vi "TCP-IP Mgr.Core.vi"(9 "Q Message Templates":T3={"Status.Q.Msg"={"Cmd"="Task", "Sub"="TCP-IP Connect Event", "Data1"=variant, "Data2"=variant}, "Rcv.Q.Msg"={"Cmd"="Task", "Sub"="TCP-IP Rcv", "Data1"=variant, "Data2"=variant}}, 10 "Config":T5={"IP"="127.0.0.1", "Port"=8500, "Listener"=FALSE, "Enable"=FALSE}, 11 "Module Config":T1={"Name"="TCP-IP Mgr", "Parent Q"=refnum, "Is Child?"=FALSE, "Index"=0, "Dirs"={"Root"=path "", "Config"=path "", "Logs"=path "", "Reports"=path "", "App Data"=path ""}, "Simulate"=FALSE, "SimCtrl"=refnum}) -> ()   [LabVIEW 2024, in "EQMF.lvlib" / "TCP-IP.lvlib"]
uses:
  TCP-IP.lvlib
  Module/Module Config.ctl
  Queues/Q.Element.ctl
  Module/Module.Working Dirs.ctl
  TCP-IP Mgr.Cluster - Q Message Templates.ctl
  TCP-IP Mgr.Config.ctl
  Module/Window/Window.Task, Action.ctl
  Strings/TextBoxLogCtrlMgr/TextBoxLogCtrlMgr.lvclass
  <vilib>/Utility/error.llb/Trim Whitespace One-Sided.vi
  Queues/Queue Utils.lvlib
  Module/Module Utils.lvlib
  Controls/Controls.lvlib
  Event Log/Event Log.lvlib
  Status/Status Utils.lvlib
panel:
  in  "Main Tab":enum32{"Operate", "Maint"}(tab)
  out "IP":string
  out "Status":string
  in  "Auto Scroll":bool
  out "Log":string
  in  "Clear":bool
  in  "Maint":bool
  out "Port":u16=8500
  in  "Show Block Diagram":bool
  in  "Leave Maint":bool
  in  "Exit":bool
  in  "Cnct Timeout":i32=1000
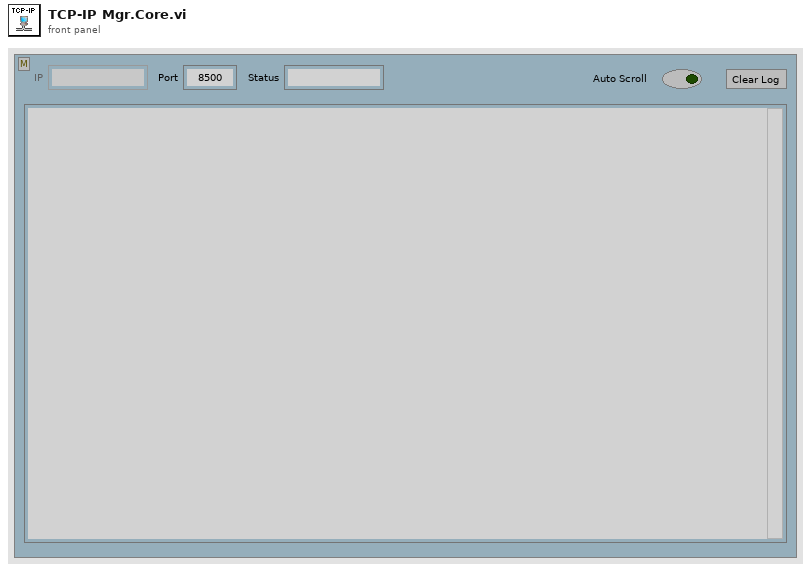
[diagram p1: front panel]
types:
  T1 = typedef "EQMF.lvlib/Module Utils.lvlib/Module Config.ctl" = cluster{"Name":string, "Parent Q":refnum<queue>, "Is Child?":bool, "Index":i32, "Dirs":T2, "Simulate":bool, "SimCtrl":refnum<vi>}
  T2 = typedef "EQMF.lvlib/Module Utils.lvlib/Module.Working Dirs.ctl" = cluster{"Root":path, "Config":path, "Logs":path, "Reports":path, "App Data":path}
  T3 = typedef "EQMF.lvlib/TCP-IP.lvlib/TCP-IP Mgr.Cluster - Q Message Templates.ctl" = cluster{"Status.Q.Msg":T4, "Rcv.Q.Msg":T4}
  T4 = typedef "EQMF.lvlib/Queue Utils.lvlib/Q.Element.ctl" = cluster{"Cmd":string, "Sub":string, "Data1":variant, "Data2":variant}
  T5 = typedef "EQMF.lvlib/TCP-IP.lvlib/TCP-IP Mgr.Config.ctl" = cluster{"IP":string, "Port":u16, "Listener":bool, "Enable":bool}
  T6 = typedef "EQMF.lvlib/Module Utils.lvlib/Module Sys Info.ctl" = cluster{"Main Q":refnum<queue>, "Exe":bool, "SW Rev":T7, "Self Ref":refnum<vi>, "Main Tab":refnum<vi>, "Pane":refnum<vi>, "Stop":cluster{"Ref":refnum<event-registration>, "Event":refnum<user-event>}, "Cfg":T1, "Services":cluster{"Name":string, "vi ref":refnum<vi>}[], "Menu Ref":refnum<k9>, "CtrlStates":refnum<class "Class.SaveCtrls.lvclass">, "Docs":cluster{"Tags":string[], "Paths":path[]}, "Log":refnum<class "Event Notification.lvclass">, "Test Controls":refnum<vi>[], "Child Modules":cluster{"Name":string, "vi ref":refnum<vi>}[], "SW Items":string[][], "AppData":refnum<class "Class.AppData.lvclass">, "Subscriptions":refnum<class "Subscription.lvclass">, "Module Config Ref":refnum<vi>}
  T7 = typedef "EQMF.lvlib/Module Utils.lvlib/Module.SW Version Info.ctl" = cluster{"AppName":string, "Company":string, "Version":string, "Description":string, "PN":string}
  T8 = typedef "EQMF.lvlib/Module Utils.lvlib/Window.Task, Action.ctl" = enum16{"Resize()", "Show Panel(Bool)", "Show Scroll Bars(Bool)", "Dock to SubPanel(SubPanel Ref)", "Undock from SubPanel()", "Return to SubPanel()", "Go To Maint Tab()", "Show Maint Tab(Bool)", "Open Block Diagram()"}
  T9 = enum16{"Top Left", "Top Right", "Bottom Left", "Bottom Right"}
  T10 = cluster{"Log":string, "Status.Q.Msg":T4, "LogMgr":refnum<class "TextBoxLogCtrlMgr.lvclass">}
  T11 = typedef "EQMF.lvlib/Status Utils.lvlib/Status.ErrorAction - Exit, Reset, Ignore.ctl" = enum16{"Exit", "Reset", "Ignore"}
  T12 = enum8{"Enabled", "Disabled", "Disabled and Grayed Out"}
  T13 = cluster{"Connected":bool, "TCPIP ID":refnum<k5>, "Config":T5, "QMsgs":T3}
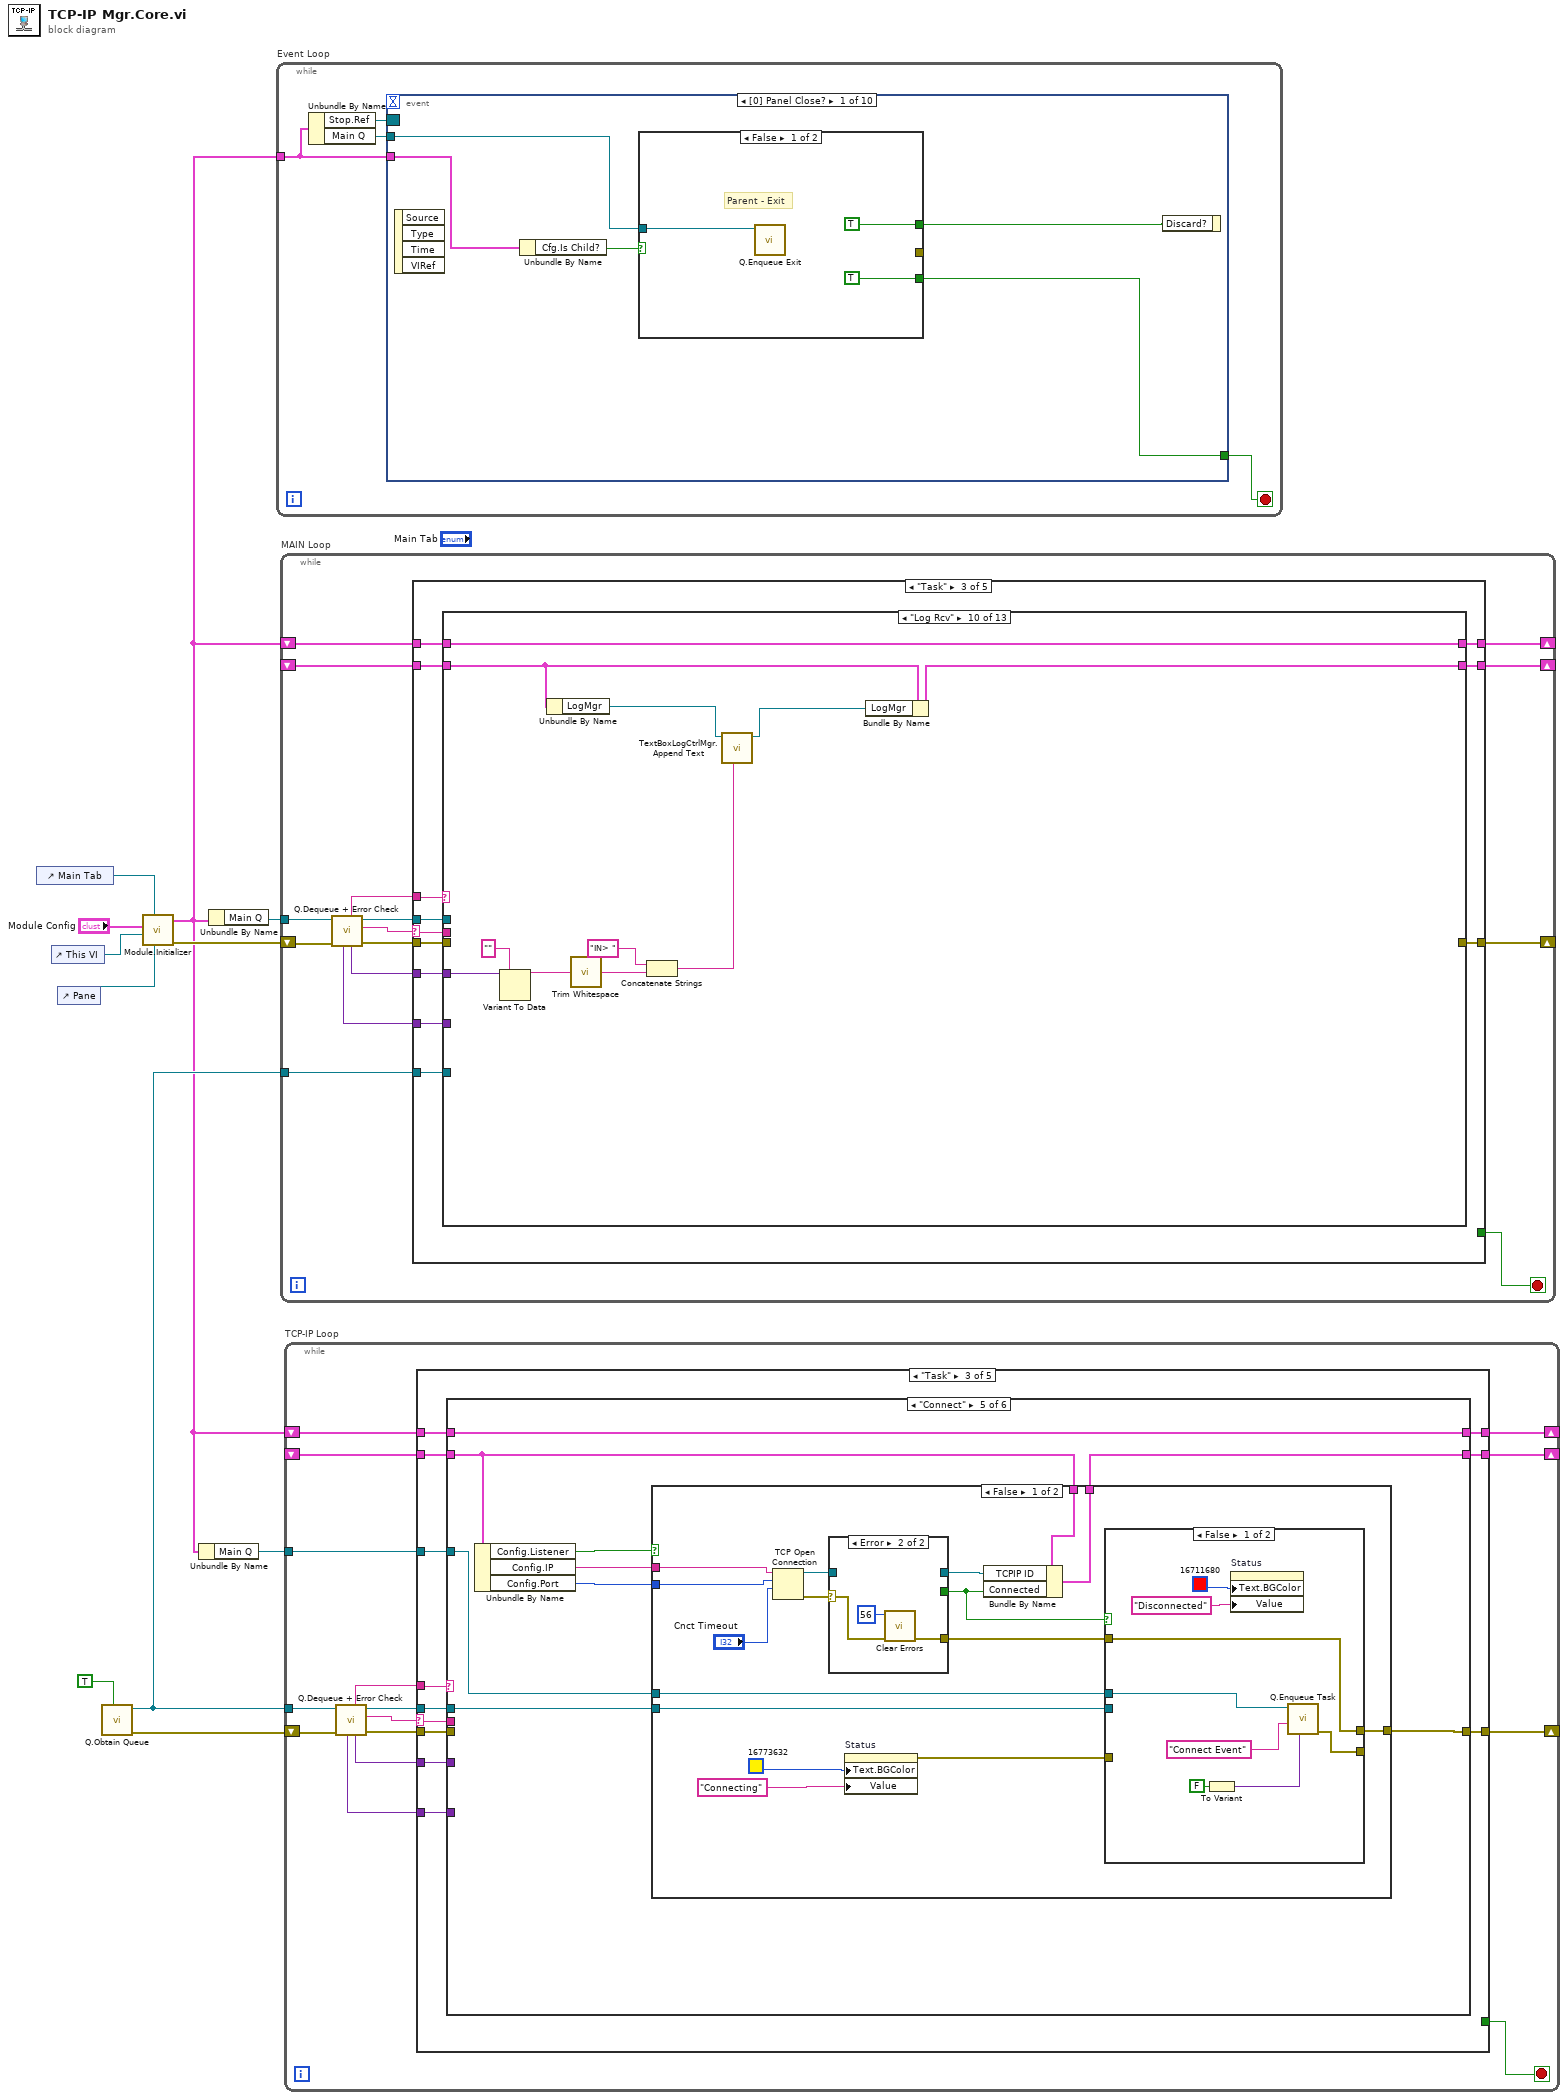
[diagram p0: block diagram]
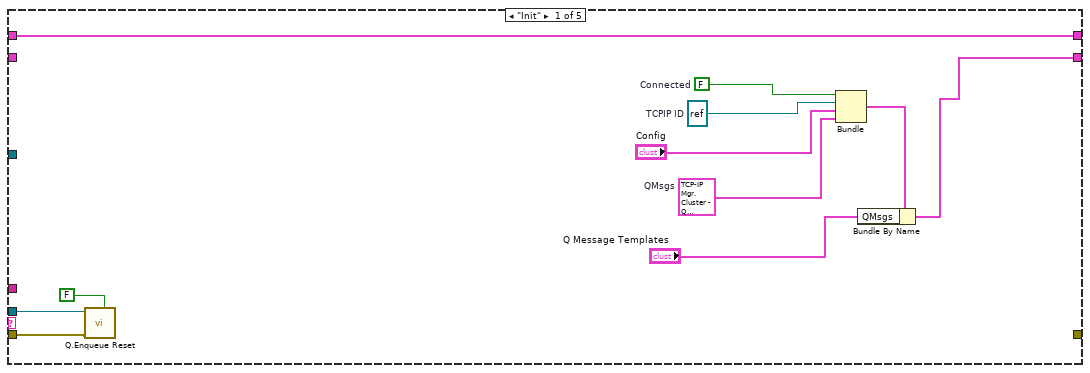
[diagram p2: hidden frame]
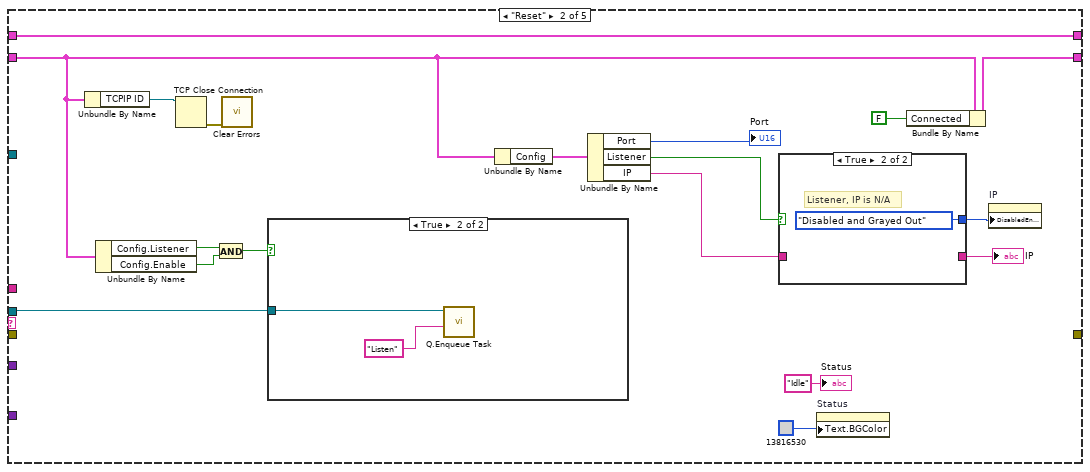
[diagram p3: hidden frame]
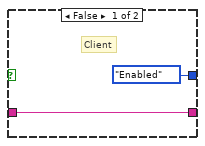
[diagram p4: hidden frame]
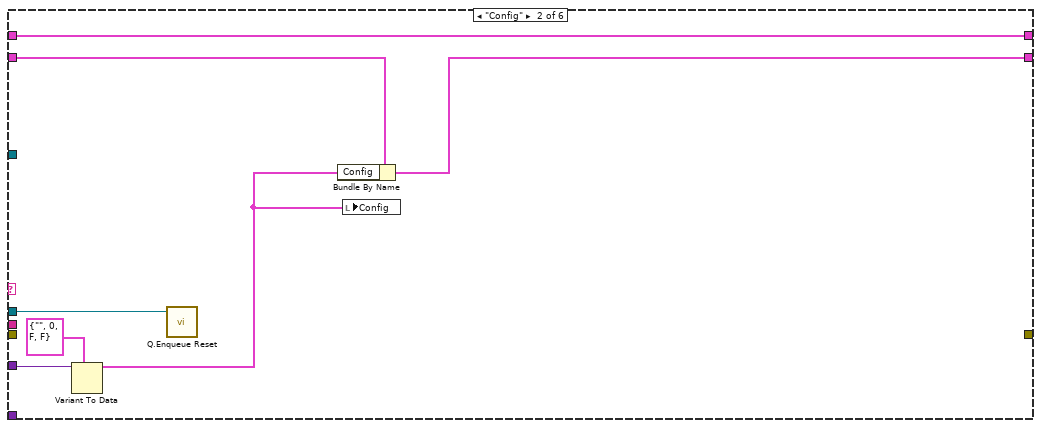
[diagram p7: hidden frame]
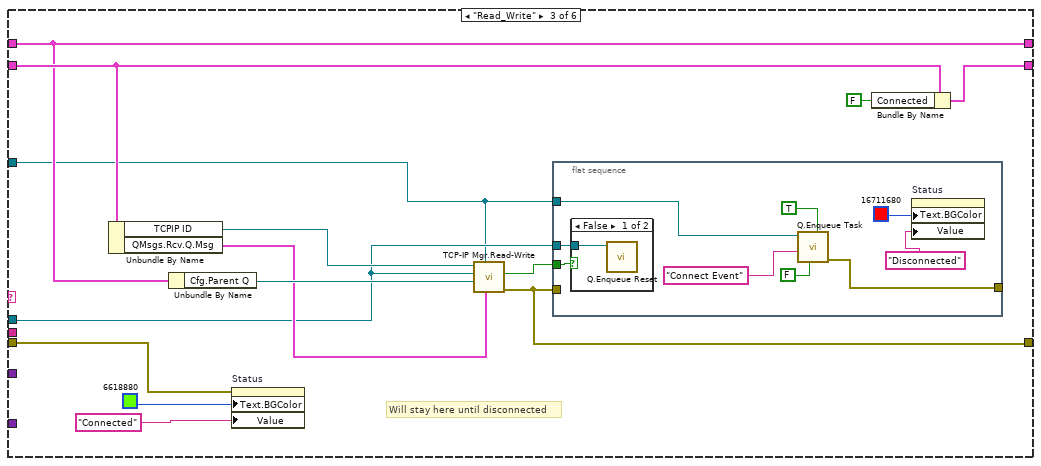
[diagram p8: hidden frame]
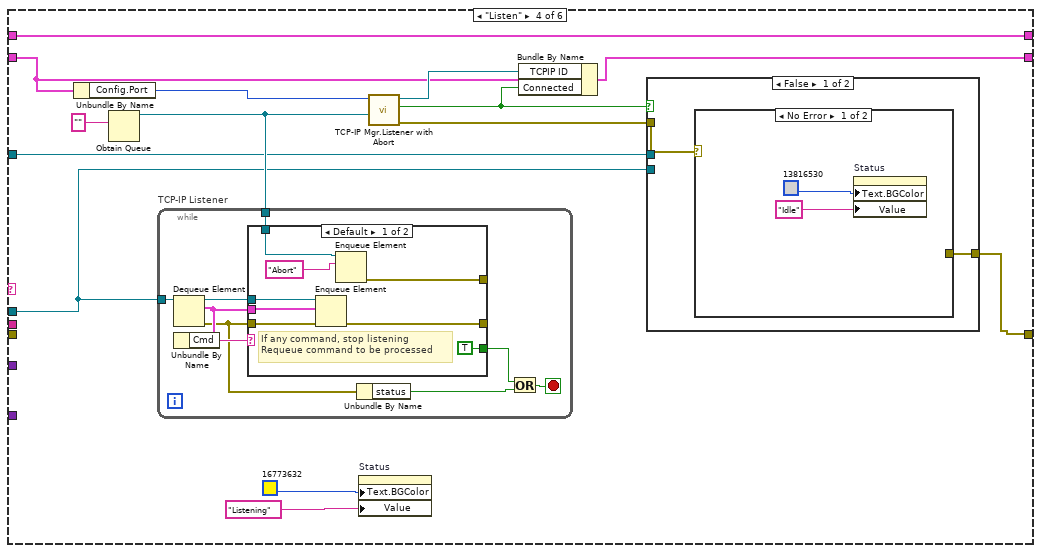
[diagram p10: hidden frame]
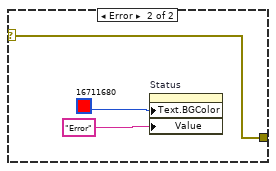
[diagram p11: hidden frame]
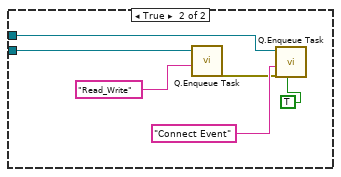
[diagram p12: hidden frame]
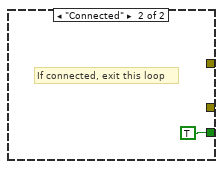
[diagram p13: hidden frame]
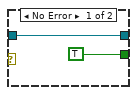
[diagram p14: hidden frame]
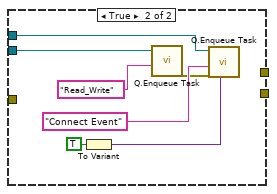
[diagram p15: hidden frame]
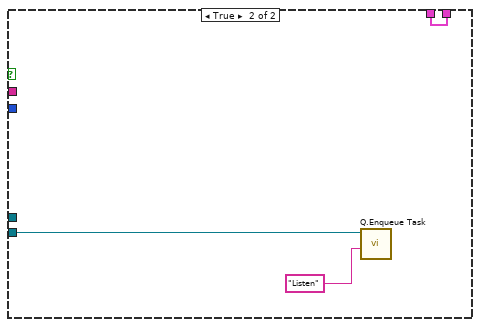
[diagram p16: hidden frame]
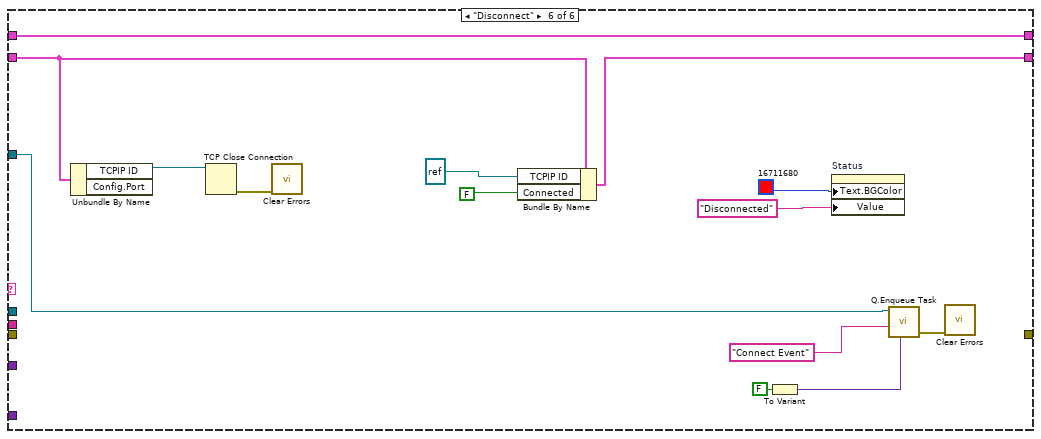
[diagram p17: hidden frame]
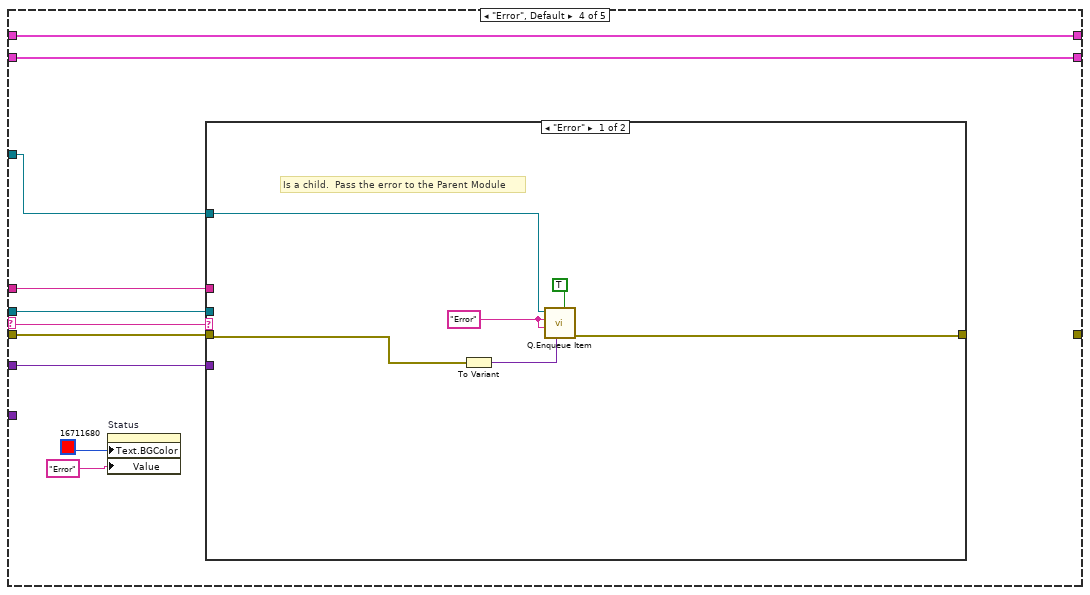
[diagram p18: hidden frame]
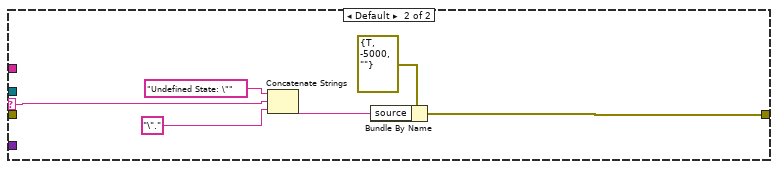
[diagram p19: hidden frame]
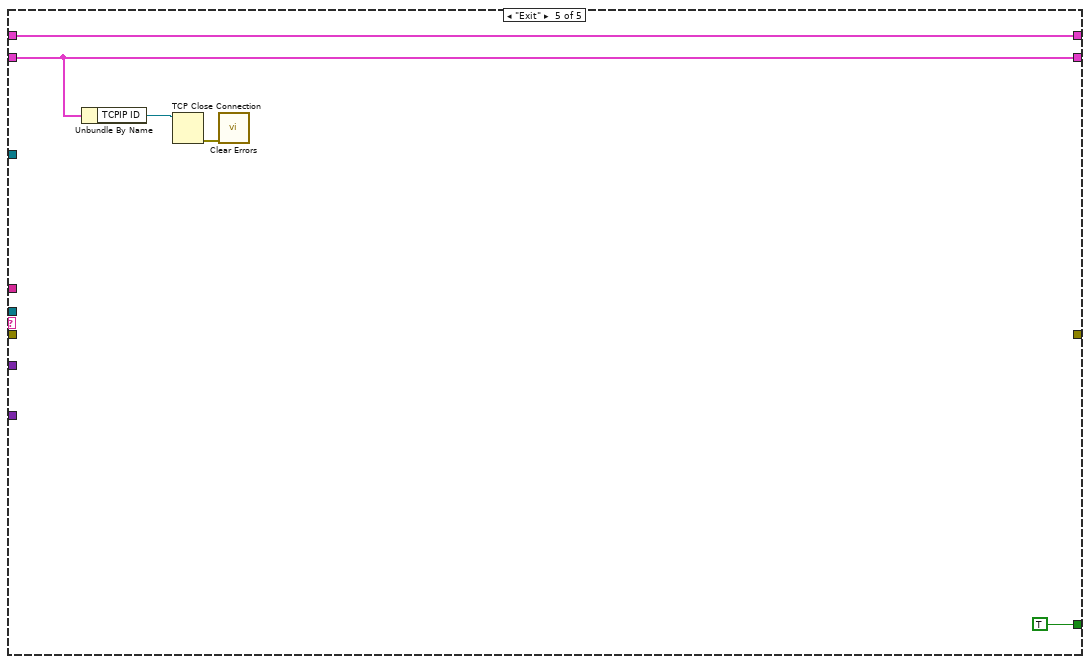
[diagram p20: hidden frame]
diagram:
  n1 = control-ref of="Main Tab"() -> (w8:refnum<vi>)
  n2 = control-ref of="This VI"() -> (w7:refnum<vi>)
  n3 = control-ref of="Pane"() -> (w1:refnum<vi>)
  n4 = call "Q.Obtain Queue.vi"("Enqueue Init"=TRUE) -> ("error out"=w4:errorcluster, "Q Out"=w5:refnum<queue>)  [unwired: 8 in, 1 out]
  n5 = call "Module.Initializer.vi"("Pane"=w1, "Main Tab"=w8, "Self Ref"=w7, "Module Config"="Module Config") -> ("error out"=w10:errorcluster, "Sys"=w2:T6)  [unwired: 6 in]
  n6 = Unbundle By Name(w2) -> ("Main Q"=w3:refnum<queue>)
  n7 = Unbundle By Name(w2) -> ("Main Q"=w9:refnum<queue>)
  n8 = while "Event Loop" {
    tunnel: w2 -> [w14]
    stop <- w15 stop-if-true
    n9 = Unbundle By Name(w14) -> ("Stop.Ref"=w13:refnum<event-registration>, "Main Q"=w12:refnum<queue>)
    n10 = event shown="[0] Panel Close?" {
      selector: w13 -> [_ _ _ _ _ _ _ _ _ _]
      dyn-events: _ -> [_ _ _ _ _ _ _ _ _ _]
      timeout: _ -> [_ _ _ _ _ _ _ _ _ _]
      tunnel: [w18 _ _ _ _ _ TRUE _ w43 TRUE] -> w15
      tunnel: w14 -> [w17 _ _ _ _ _ _ _ _ _]
      tunnel: w12 -> [w20 w30 w32 w34 w35 w38 w39 _ w42 _]
      event Panel Close? {
        n11 = event-data() -> ()  [unwired: 1 in, 4 out]
        n12 = Unbundle By Name(w17) -> ("Cfg.Is Child?"=w16:bool)
        n13 = case shown="False" w16 {
          tunnel: w20 -> [w23 w26]
          tunnel: [TRUE TRUE] -> w19
          tunnel: [TRUE FALSE] -> w18
          tunnel: [_ w24] -> _
          frame False {
            # "Parent - Exit"
            n14 = call "Q.Enqueue Exit.vi"("Q In"=w23) -> ()  [unwired: 9 in, 2 out]
          }
          frame True {
            # "Child - Hide Panel"
            n15 = call "Module.Window, Q Task.vi"("Action"=Window.Task,_Action."Show Panel(Bool)", "Q In"=w26) -> ("error out"=w24:errorcluster)  [unwired: 8 in, 1 out]
          }
        }
        n16 = event-data("Discard?"=w19) -> ()  [unwired: 1 in, 1 out]
      }
      event Panel Resize {
        n17 = event-data() -> ()  [unwired: 1 in, 8 out]
        n18 = call "Module.Window, Q Task.vi"("Action"=Window.Task,_Action."Resize()", "Q In"=w30) -> ()  [unwired: 8 in, 2 out]
      }
      event "Show Block Diagram": Value Change {
        n19 = event-data() -> ()  [unwired: 1 in, 6 out]
        n20 = call "Module.Window, Q Task.vi"("Action"=Window.Task,_Action."Open Block Diagram()", "Q In"=w32) -> ()  [unwired: 8 in, 2 out]
      }
      event "Maint": Value Change {
        n21 = event-data() -> ()  [unwired: 1 in, 6 out]
        n22 = call "Module.Window, Q Task.vi"("Action"=Window.Task,_Action."Go To Maint Tab()", "Q In"=w34) -> ()  [unwired: 8 in, 2 out]
      }
      event "Auto Scroll": Value Change {
        n23 = event-data() -> ()  [unwired: 1 in, 6 out]
        n24 = call "Q.Enqueue Task.vi"("Task Name"="Set  Auto Scroll", "Q In"=w35) -> ()  [unwired: 8 in, 2 out]
      }
      event "Clear": Value Change {
        n25 = event-data() -> ()  [unwired: 1 in, 6 out]
        n26 = call "Q.Enqueue Task.vi"("Task Name"="Clear Log", "Q In"=w38) -> ()  [unwired: 8 in, 2 out]
      }
      event "Exit": Value Change {
        n27 = event-data() -> ()  [unwired: 1 in, 6 out]
        n28 = call "Q.Enqueue Exit.vi"("Q In"=w39) -> ()  [unwired: 9 in, 2 out]
      }
      event "Leave Maint": Value Change {
        n29 = event-data() -> ()  [unwired: 1 in, 6 out]
        n30 = local write "Main Tab"(0) -> ()
      }
      event Menu Selection (User) {
        n31 = event-data() -> ("ItemTag"=w44:string)  [unwired: 1 in, 6 out]
        n32 = case shown="\"Exit\"" w44 {
          tunnel: [_ TRUE] -> w43
          tunnel: w42 -> [_ w45]
          frame "False", Default {
          }
          frame "Exit" {
            n33 = call "Q.Enqueue Exit.vi"("Q In"=w45) -> ()  [unwired: 9 in, 2 out]
          }
        }
      }
      event User Event {
        n34 = event-data() -> ()  [unwired: 1 in, 5 out]
      }
    }
  }
  n35 = while "MAIN Loop" {
    shift-right: [w58] -> _
    shift-left: w10 -> [w56]
    shift-right: [w59] -> _
    shift-left: _ -> [w62]
    shift-right: [w60] -> _
    shift-left: w2 -> [w61]
    tunnel: w9 -> [w55]
    tunnel: w5 -> [w48]
    stop <- w49 stop-if-true
    n36 = call "Q.Dequeue + Error Check.vi"("Error In"=w56, "Q In"=w55) -> ("error out"=w57:errorcluster, "Cmd"=w54:string, "Q Out"=w53:refnum<queue>, "Data1"=w52:variant, "Sub"=w50:string, "Data2"=w51:variant)  [unwired: 4 in]
    n37 = case shown="\"Task\"" w54 {
      selector: w54 -> [_ _ w93 w242 _]
      tunnel: w62 -> [_ w85 w102 w247 w291]
      tunnel: w61 -> [w69 w91 w103 w239 w293]
      tunnel: [w69 w91 w101 w239 w293] -> w60
      tunnel: [w65 w84 w100 w247 w291] -> w59
      tunnel: [_ _ w94 _ w295] -> w58
      tunnel: w57 -> [w75 _ w96 w241 w294]
      tunnel: w53 -> [w76 w88 w97 w243 _]
      tunnel: w52 -> [_ _ w98 w240 _]
      tunnel: w51 -> [_ _ w95 _ _]
      tunnel: w50 -> [_ _ w99 w244 _]
      tunnel: [_ _ _ _ TRUE] -> w49
      tunnel: w48 -> [_ w86 w92 _ w289]
      frame "Init" {
        w63 = refnum<class "TextBoxLogCtrlMgr.lvclass"> refnum  # LogMgr
        w67 = T4 {"Cmd"="", "Sub"="", "Data1"=variant, "Data2"=variant}  # Status.Q.Msg
        w70 = ""  # Log
        # "Only allow \"Show block diagram\" in development"
        n38 = Unbundle By Name(w69) -> ("Exe"=w73:bool)
        n39 = call "Q.Enqueue Reset.vi"("Top of Q(T)"=FALSE ("Flush Q"), "Error In"=w75, "Q In"=w76) -> ()  [unwired: 7 in, 2 out]
        n40 = Not(x=w73) -> (.not. x?=w72:bool)
        n41 = local write "Auto Scroll"(TRUE ("Auto Scroll")) -> ()
        n42 = property on="Show Block Diagram" class="Bool"("Visible"=w72) -> ()  [unwired: 2 in, 2 out]
        n43 = property on="Maint" class="Bool"("Visible"=w72) -> ()  [unwired: 2 in, 2 out]
        n44 = local read "Q Message Templates"() -> (w68:T3)
        n45 = Unbundle By Name(w68) -> ("Status.Q.Msg"=w64:T4)
        n46 = Bundle("Log"=w70, "Status.Q.Msg"=w67, "LogMgr"=w63) -> (w66:T10)  [unwired: 1 in]
        n47 = Bundle By Name(cluster=w66, "Status.Q.Msg"=w64) -> (w65:T10)
      }
      frame "Reset" {
        n48 = call "Q.Enqueue Reset.vi"("Q In"=w86) -> ()  [unwired: 9 in, 2 out]
        n49 = call "Q.Enqueue Task.vi"("Task Name"="Clear Log", "Q In"=w88) -> ()  [unwired: 8 in, 2 out]
        n50 = control-ref of="Log"() -> (w79:refnum<vi>)
        n51 = Unbundle By Name(w85) -> ("LogMgr"=w83:refnum<class "TextBoxLogCtrlMgr.lvclass">)
        n52 = property on="Log" class="Str"("Text.Scroll Position"=u32 0) -> ()  [unwired: 2 in, 2 out]
        n53 = call "TextBoxLogCtrlMgr.Initialize.vi"("DataStamp"=FALSE, "TimeStamp"=TRUE, "MaxLen"=10000, "Auto Scroll"="Auto Scroll", "CtrlRef"=w79, "TextBoxLogCtrlMgr in"=w83) -> ("TextBoxLogCtrlMgr out"=w82:refnum<class "TextBoxLogCtrlMgr.lvclass">)  [unwired: 4 in, 1 out]
        n54 = Bundle By Name(cluster=w85, "LogMgr"=w82) -> (w84:T10)
        "Log" <- "" ("Log")
      }
      frame "Task" {
        n55 = case shown="\"Log Rcv\"" w99 {
          selector: w99 -> [w108 _ _ _ _ _ _ _ _ _ _ _ _]
          tunnel: w103 -> [w109 w116 w161 w166 w171 w176 w181 w188 w204 w215 w225 w230 w236]
          tunnel: w102 -> [w110 w117 w160 w165 w170 w175 w180 w190 w201 w212 w222 w229 w235]
          tunnel: [w109 w116 w161 w166 w171 w176 w181 w188 w204 w215 w225 w230 w236] -> w101
          tunnel: [w110 w117 w160 w165 w170 w175 w180 w190 w200 w211 w221 w228 w234] -> w100
          tunnel: w98 -> [w107 _ w159 w164 w169 w174 w179 w191 w202 w213 w223 _ _]
          tunnel: w97 -> [_ _ _ _ _ _ _ _ _ _ _ _ _]
          tunnel: w96 -> [w105 _ _ _ _ _ _ _ _ _ _ _ _]
          tunnel: w95 -> [w106 _ _ _ _ _ _ _ _ _ _ _ _]
          tunnel: [w104 _ _ _ _ _ _ _ _ _ _ _ _] -> w94
          tunnel: w93 -> [_ _ _ _ _ _ _ _ _ _ _ _ _]
          tunnel: w92 -> [_ _ w158 w163 w168 w173 w178 _ _ _ _ _ _]
          frame Default {
            n56 = call "Module.Default Tasks.vi"("Sys"=w109, "error in"=w105, "Data2"=w106, "Data1"=w107, "Sub"=w108) -> ("error out"=w104:errorcluster)  [unwired: 5 in, 1 out]
          }
          frame "Resize" {
            n57 = control-ref of="Clear"() -> (w113:refnum<vi>)
            n58 = Unbundle By Name(w116) -> ("Main Tab"=w115:refnum<vi>)
            n59 = control-ref of="Auto Scroll"() -> (w112:refnum<vi>)
            n60 = control-ref of="IP"() -> (w111:refnum<vi>)
            n61 = control-ref of="Log"() -> (w114:refnum<vi>)
            n62 = while {
              tunnel: w115 -> [w122]
              tunnel: w114 -> [w121]
              tunnel: w113 -> [w120]
              tunnel: w112 -> [w119]
              tunnel: w111 -> [w118]
              i -> [w124]
              stop <- w123 stop-if-true
              n63 = case shown="0" w124 {
                tunnel: [_ _ _ TRUE] -> w123
                tunnel: w122 -> [w128 _ w147 w155]
                tunnel: w121 -> [_ _ w141 w154]
                tunnel: w120 -> [w126 w132 _ w153]
                tunnel: w119 -> [_ w131 _ w152]
                tunnel: [_ _ _ w150] -> _
                tunnel: w118 -> [_ _ _ _]
                frame 0 {
                  # "Clear Log in top rt corner"
                  n64 = call "Resize.Align Ctrl within Tab Ctrl.vi"("Child Ref Pos"=T9."Top Right", "dY"=15 ("dX"), "Parent Ref Pos"=T9."Top Right", "dX"=10, "Child Ctrl"=w126, "Parent Tab Ctrl"=w128) -> ()  [unwired: 3 in, 3 out]
                }
                frame 1 {
                  # "Auto Scroll is left of Clear Log"
                  n65 = call "Resize.Align Ctrl with Ctrl.vi"("Move Ctrl Ref Location"=T9."Top Right" ("Child Ref Pos"), "dY"=-5 ("dX"), "Ref Ctrl Corner"=T9."Top Left" ("Parent Ref Pos"), "dX"=20, "Move Ctrl"=w131, "Ref Ctrl"=w132) -> ()  [unwired: 3 in, 3 out]
                }
                frame 2 {
                  # "Center Log in Tab Control"
                  n66 = property class="TabCtl"(reference=w147) -> ("Height"=w146:u32, "Width"=w145:u32)  [unwired: 1 in, 2 out]
                  n67 = Subtract(x=w146, y=u32 65) -> (x-y=w137:u32)
                  n68 = Subtract(x=w145, y=u32 20) -> (x-y=w143:u32)
                  n69 = property class="Str"(reference=w141, "Height"=w137, "Width"=w143) -> (reference out=w142:refnum<vi>)  [unwired: 1 in, 1 out]
                  n70 = call "Resize.Align Ctrl within Tab Ctrl.vi"("Child Ref Pos"=T9."Top Left", "dY"=u32 50 ("y"), "Parent Ref Pos"=T9."Top Left", "dX"=u32 10 ("y"), "Child Ctrl"=w142, "Parent Tab Ctrl"=w147) -> ()  [unwired: 3 in, 3 out]
                }
                frame Default {
                  # "Done"
                  n71 = Build Array(w155, w154, w153, w152) -> (w151:refnum<vi>[])
                  n72 = Close Reference(reference=w151) -> (error out=w150:errorcluster)  [unwired: 1 in]
                }
              }
            }
          }
          frame "Config" {
            n73 = call "Q.Enqueue Task.vi"("Data1"=w159, "Task Name"="Config", "Q In"=w158) -> ()  [unwired: 7 in, 2 out]
          }
          frame "Connect" {
            n74 = call "Q.Enqueue Task.vi"("Data1"=w164, "Task Name"="Connect", "Q In"=w163) -> ()  [unwired: 7 in, 2 out]
          }
          frame "Send" {
            n75 = call "Q.Enqueue Task.vi"("Data1"=w169, "Task Name"="Send", "Q In"=w168) -> ()  [unwired: 7 in, 2 out]
          }
          frame "Disconnect" {
            n76 = call "Q.Enqueue Task.vi"("Data1"=w174, "Task Name"="Disconnect", "Q In"=w173) -> ()  [unwired: 7 in, 2 out]
          }
          frame "Listen" {
            n77 = call "Q.Enqueue Task.vi"("Data1"=w179, "Task Name"="Listen", "Q In"=w178) -> ()  [unwired: 7 in, 2 out]
          }
          frame "Connect Event" {
            n78 = Variant To Data(type=FALSE, Variant=w191) -> (data=w186:bool)  [unwired: 1 in, 1 out]
            n79 = Unbundle By Name(w188) -> ("Cfg.Parent Q"=w187:refnum<queue>)
            n80 = Unbundle By Name(w190) -> ("Status.Q.Msg"=w189:T4)
            n81 = case shown="False" w186 {
              tunnel: ["STATE> Connected" ("Status") "STATE> Disconnected" ("Status")] -> w182
              frame True {
              }
              frame False {
              }
            }
            n82 = Unbundle By Name(w189) -> ("Cmd"=w193:string, "Sub"=w192:string)
            n83 = call "Q.Enqueue Item.vi"("Data1"=w186, "Sub"=w192, "Cmd"=w193, "Q In"=w187) -> ("Q Out"=w184:refnum<queue>)  [unwired: 6 in, 1 out]
            n84 = call "Q.Enqueue Task.vi"("Top of Q"=TRUE, "Data1"=w182, "Task Name"="Log Msg", "Q In"=w184) -> ()  [unwired: 6 in, 2 out]
          }
          frame "Log Msg" {
            n85 = Variant To Data(type="", Variant=w202) -> (data=w197:string)  [unwired: 1 in, 1 out]
            n86 = Unbundle By Name(w201) -> ("LogMgr"=w199:refnum<class "TextBoxLogCtrlMgr.lvclass">)
            n87 = call "TextBoxLogCtrlMgr.Append Text.vi"("Text In"=w197, "TextBoxLogCtrlMgr in"=w199) -> ("TextBoxLogCtrlMgr out"=w198:refnum<class "TextBoxLogCtrlMgr.lvclass">)  [unwired: 8 in, 1 out]
            n88 = Bundle By Name(cluster=w201, "LogMgr"=w198) -> (w200:T10)
          }
          frame "Log Rcv" {
            n89 = Variant To Data(type="", Variant=w213) -> (data=w205:string)  [unwired: 1 in, 1 out]
            n90 = Unbundle By Name(w212) -> ("LogMgr"=w210:refnum<class "TextBoxLogCtrlMgr.lvclass">)
            n91 = call <vilib>:"Trim Whitespace.vi"("string"=w205) -> ("trimmed string"=w206:string)  [unwired: 1 in]
            n92 = Concatenate Strings("IN> ", w206) -> (w207:string)
            n93 = call "TextBoxLogCtrlMgr.Append Text.vi"("Text In"=w207, "TextBoxLogCtrlMgr in"=w210) -> ("TextBoxLogCtrlMgr out"=w209:refnum<class "TextBoxLogCtrlMgr.lvclass">)  [unwired: 8 in, 1 out]
            n94 = Bundle By Name(cluster=w212, "LogMgr"=w209) -> (w211:T10)
          }
          frame "Log Send" {
            n95 = Variant To Data(type="", Variant=w223) -> (data=w217:string)  [unwired: 1 in, 1 out]
            n96 = Unbundle By Name(w222) -> ("LogMgr"=w220:refnum<class "TextBoxLogCtrlMgr.lvclass">)
            n97 = Concatenate Strings("OUT> ", w217) -> (w216:string)
            n98 = call "TextBoxLogCtrlMgr.Append Text.vi"("Text In"=w216, "TextBoxLogCtrlMgr in"=w220) -> ("TextBoxLogCtrlMgr out"=w219:refnum<class "TextBoxLogCtrlMgr.lvclass">)  [unwired: 8 in, 1 out]
            n99 = Bundle By Name(cluster=w222, "LogMgr"=w219) -> (w221:T10)
          }
          frame "Clear Log" {
            n100 = Unbundle By Name(w229) -> ("LogMgr"=w226:refnum<class "TextBoxLogCtrlMgr.lvclass">)
            n101 = call "TextBoxLogCtrlMgr.Clear.vi"("TextBoxLogCtrlMgr in"=w226) -> ("TextBoxLogCtrlMgr out"=w227:refnum<class "TextBoxLogCtrlMgr.lvclass">)  [unwired: 9 in, 1 out]
            n102 = Bundle By Name(cluster=w229, "LogMgr"=w227) -> (w228:T10)
          }
          frame "Set  Auto Scroll" {
            n103 = Unbundle By Name(w235) -> ("LogMgr"=w232:refnum<class "TextBoxLogCtrlMgr.lvclass">)
            n104 = local read "Auto Scroll"() -> (w231:bool)
            n105 = call "TextBoxLogCtrlMgr.Set Auto Scroll.vi"("Auto Scroll"=w231, "TextBoxLogCtrlMgr in"=w232) -> ("TextBoxLogCtrlMgr out"=w233:refnum<class "TextBoxLogCtrlMgr.lvclass">)  [unwired: 8 in, 1 out]
            n106 = Bundle By Name(cluster=w235, "LogMgr"=w233) -> (w234:T10)
          }
        }
      }
      frame "Error", Default {
        n107 = Unbundle By Name(w239) -> ("Cfg.Is Child?"=w246:bool, "Cfg.Parent Q"=w245:refnum<queue>)
        n108 = property on="Status" class="Str"("Text.BGColor"=u32 16711680, "Value"="Error" ("Status")) -> ()  [unwired: 2 in, 2 out]
        n109 = case shown="\"Error\"" w242 {
          selector: w242 -> [_ w280]
          tunnel: [w250 w281] -> _
          tunnel: w240 -> [w254 _]
          tunnel: w241 -> [w252 _]
          tunnel: w244 -> [w253 _]
          tunnel: w243 -> [w251 _]
          tunnel: w246 -> [w249 _]
          tunnel: w245 -> [w248 _]
          frame "Error" {
            n110 = case shown="False" w249 {
              tunnel: w254 -> [w263 _]
              tunnel: w253 -> [w262 _]
              tunnel: w252 -> [w261 w276]
              tunnel: w251 -> [w259 _]
              tunnel: [w257 w274] -> w250
              tunnel: w248 -> [_ w279]
              frame False {
                # "Is running as Parent or Individual Module\nHandle Error Here"
                n111 = case shown="\"Error\"" w262 {
                  tunnel: w263 -> [_ w273]
                  tunnel: w261 -> [w269 _]
                  tunnel: [w269 w271] -> w256
                  tunnel: w259 -> [w268 w270]
                  tunnel: [w268 w270] -> w258
                  frame Default {
                  }
                  frame "Error" {
                    n112 = Variant To Data(type=errorcluster {"status"=FALSE, "code"=0, "source"=""} ("error constant"), Variant=w273) -> (data=w271:errorcluster)  [unwired: 1 in, 1 out]
                  }
                }
                n113 = call "Status.Dialog - Error Message.vi"("error in"=w256) -> ("Selection"=w260:T11)
                n114 = call "Event Log.Record Event.vi"("error in"=w256) -> ("error out"=w255:errorcluster)  [unwired: 10 in]
                n115 = case shown="\"Exit\", Default" w260 {
                  tunnel: w258 -> [w265 _ w267]
                  tunnel: [w264 _ w266] -> w257
                  tunnel: w255 -> [_ _ _]
                  frame "Exit", Default {
                    n116 = call "Q.Enqueue Exit.vi"("Q In"=w265) -> ("error out"=w264:errorcluster)  [unwired: 9 in, 1 out]
                  }
                  frame "Ignore" {
                  }
                  frame "Reset" {
                    n117 = call "Q.Enqueue Reset.vi"("Q In"=w267) -> ("error out"=w266:errorcluster)  [unwired: 9 in, 1 out]
                  }
                }
              }
              frame True {
                w277 = "Error" ("Cmd")
                # "Is a child.  Pass the error to the Parent Module"
                n118 = To Variant(anything=w276) -> (Variant=w275:variant)
                n119 = call "Q.Enqueue Item.vi"("Top of Q"=TRUE, "Data1"=w275, "Sub"=w277, "Cmd"=w277, "Q In"=w279) -> ("error out"=w274:errorcluster)  [unwired: 5 in, 1 out]
              }
            }
          }
          frame Default {
            n120 = Concatenate Strings("Undefined State: \"", w280, "\".") -> (w282:string)
            n121 = Bundle By Name(cluster=errorcluster {"status"=TRUE, "code"=-5000, "source"=""} ("error constant"), "source"=w282) -> (w281:errorcluster)
          }
        }
      }
      frame "Exit" {
        n122 = Flush Queue(queue=w289) -> (queue out=w290:refnum<queue>)  [unwired: 1 in, 2 out]
        n123 = call "Q.Enqueue Task.vi"("Top of Q"=TRUE, "Task Name"="Disconnect", "Q In"=w290) -> ("Q Out"=w287:refnum<queue>)  [unwired: 7 in, 1 out]
        n124 = call "Q.Enqueue Exit.vi"("Q In"=w287) -> ()  [unwired: 9 in, 2 out]
        n125 = call "Module.Destructor.vi"("error in"=w294, "Sys"=w293) -> ("error out"=w295:errorcluster)  [unwired: 9 in]
      }
    }
  }
  n126 = while "TCP-IP Loop" {
    shift-right: [w306] -> _
    shift-left: w4 -> [w304]
    shift-right: [w307] -> _
    shift-left: _ -> [w310]
    shift-right: [w308] -> _
    shift-left: w2 -> [w309]
    tunnel: w5 -> [w303]
    tunnel: w3 -> [w296]
    stop <- w297 stop-if-true
    n127 = call "Q.Dequeue + Error Check.vi"("Error In"=w304, "Q In"=w303) -> ("error out"=w305:errorcluster, "Cmd"=w302:string, "Q Out"=w301:refnum<queue>, "Data1"=w300:variant, "Sub"=w298:string, "Data2"=w299:variant)  [unwired: 4 in]
    n128 = case shown="\"Task\"" w302 {
      selector: w302 -> [_ _ w346 w503 _]
      tunnel: w310 -> [_ w325 w355 w506 w519]
      tunnel: w309 -> [w313 w339 w356 w500 w523]
      tunnel: [w313 w339 w354 w500 w523] -> w308
      tunnel: [w315 w338 w353 w506 w519] -> w307
      tunnel: [_ _ w347 _ _] -> w306
      tunnel: w305 -> [w320 _ w349 w502 _]
      tunnel: w301 -> [w321 w334 w350 w504 _]
      tunnel: w300 -> [_ _ w351 w501 _]
      tunnel: w299 -> [_ _ w348 _ _]
      tunnel: w298 -> [_ _ w352 w505 _]
      tunnel: [_ _ _ _ TRUE] -> w297
      tunnel: w296 -> [_ _ w345 w497 _]
      frame "Init" {
        w314 = T3 {"Status.Q.Msg"={"Cmd"="Task", "Sub"="TCP-IP Connect Event", "Data1"=variant, "Data2"=variant}, "Rcv.Q.Msg"={"Cmd"="Task", "Sub"="TCP-IP Rcv", "Data1"=variant, "Data2"=variant}}  # QMsgs
        w317 = refnum<k5> refnum  # TCPIP ID
        w318 = FALSE  # Connected
        n129 = call "Q.Enqueue Reset.vi"("Top of Q(T)"=FALSE ("Flush Q"), "Error In"=w320, "Q In"=w321) -> ()  [unwired: 7 in, 2 out]
        n130 = Bundle("Connected"=w318, "TCPIP ID"=w317, "Config"="Config", "QMsgs"=w314) -> (w316:T13)  [unwired: 1 in]
        n131 = Bundle By Name(cluster=w316, "QMsgs"="Q Message Templates") -> (w315:T13)
      }
      frame "Reset" {
        n132 = Unbundle By Name(w325) -> ("TCPIP ID"=w336:refnum<k5>)
        n133 = Unbundle By Name(w325) -> ("Config.Listener"=w331:bool, "Config.Enable"=w322:bool)
        n134 = TCP Close Connection(connection ID=w336) -> (error out=w337:errorcluster)  [unwired: 2 in, 1 out]
        n135 = And(x=w331, y=w322) -> (x .and. y?=w330:bool)
        n136 = call <vilib>:"Clear Errors.vi"("error in (no error)"=w337) -> ()  [unwired: 5 in, 2 out]
        n137 = case shown="True" w330 {
          tunnel: w334 -> [_ w343]
          frame False {
          }
          frame True {
            n138 = call "Q.Enqueue Task.vi"("Task Name"="Listen", "Q In"=w343) -> ()  [unwired: 8 in, 2 out]
          }
        }
        n139 = Unbundle By Name(w325) -> ("Config"=w324:T5)
        n140 = Unbundle By Name(w324) -> ("Port"=→"Port":u16, "Listener"=w329:bool, "IP"=w327:string)
        n141 = case shown="True" w329 {
          tunnel: [T12."Enabled" ("Disabled") T12."Disabled and Grayed Out" ("Disabled")] -> w328
          tunnel: w327 -> [w340 _]
          tunnel: [w340 _] -> w326
          frame False {
            # "Client"
          }
          frame True {
            # "Listener, IP is N/A"
          }
        }
        "IP" <- w326
        n142 = property on="Status" class="Str"("Text.BGColor"=u32 13816530) -> ()  [unwired: 2 in, 2 out]
        n143 = Bundle By Name(cluster=w325, "Connected"=FALSE ("Running")) -> (w338:T13)
        n144 = property on="IP" class="Str"("DisabledEnum"=w328) -> ()  [unwired: 2 in, 2 out]
        "Status" <- "Idle" ("Status")
      }
      frame "Task" {
        n145 = case shown="\"Connect\"" w352 {
          tunnel: w356 -> [w357 w365 w374 w403 w443 w496]
          tunnel: w355 -> [w358 w362 w375 w394 w440 w495]
          tunnel: [w357 w365 w374 w403 w443 w496] -> w354
          tunnel: [w358 w361 w378 w393 w441 w494] -> w353
          tunnel: w351 -> [_ w363 _ _ _ _]
          tunnel: w350 -> [_ w360 w368 w395 w439 _]
          tunnel: w349 -> [_ _ w370 _ _ _]
          tunnel: w348 -> [_ _ _ _ _ _]
          tunnel: [_ _ w376 w396 w442 _] -> w347
          tunnel: w346 -> [_ _ _ _ _ _]
          tunnel: w345 -> [_ _ w367 w390 w438 w484]
          frame Default {
            # "Do Nothing"
          }
          frame "Config" {
            n146 = Variant To Data(type=T5 {"IP"="", "Port"=0, "Listener"=FALSE, "Enable"=FALSE} ("Config"), Variant=w363) -> (data=w359:T5)  [unwired: 1 in, 1 out]
            n147 = call "Q.Enqueue Reset.vi"("Q In"=w360) -> ()  [unwired: 9 in, 2 out]
            n148 = Bundle By Name(cluster=w362, "Config"=w359) -> (w361:T13)
            n149 = local write "Config"(w359) -> ()
          }
          frame "Read_Write" {
            # "Will stay here until disconnected"
            n150 = Unbundle By Name(w375) -> ("TCPIP ID"=w377:refnum<k5>, "QMsgs.Rcv.Q.Msg"=w372:T4)
            n151 = Unbundle By Name(w374) -> ("Cfg.Parent Q"=w373:refnum<queue>)
            n152 = property on="Status" class="Str"(error in=w370, "Text.BGColor"=u32 6618880, "Value"="Connected" ("Status")) -> ()  [unwired: 1 in, 2 out]
            n153 = call "TCP-IP Mgr.Read-Write.vi"("Rcv Q.Element"=w372, "Q Local"=w367, "Q.Rcv"=w373, "Q Send"=w368, "TCPIP ID"=w377) -> ("error out"=w376:errorcluster, "Disconnect/Exit"=w366:bool)  [unwired: 5 in]
            n154 = flat-sequence {
              tunnel: w367 -> [w385]
              tunnel: w376 -> [_]
              tunnel: w368 -> [w384]
              tunnel: [w381] -> _
              tunnel: w366 -> [w380]
              frame #0 {
                n155 = case shown="False" w380 {
                  tunnel: w384 -> [w389 _]
                  frame False {
                    n156 = call "Q.Enqueue Reset.vi"("Q In"=w389) -> ()  [unwired: 9 in, 2 out]
                  }
                  frame True {
                  }
                }
                n157 = call "Q.Enqueue Task.vi"("Top of Q"=TRUE, "Data1"=FALSE, "Task Name"="Connect Event" ("Cmd"), "Q In"=w385) -> ("error out"=w381:errorcluster)  [unwired: 6 in, 1 out]
                n158 = property on="Status" class="Str"("Text.BGColor"=u32 16711680, "Value"="Disconnected" ("Status")) -> ()  [unwired: 2 in, 2 out]
              }
            }
            n159 = Bundle By Name(cluster=w375, "Connected"=FALSE) -> (w378:T13)
          }
          frame "Listen" {
            n160 = Unbundle By Name(w394) -> ("Config.Port"=w400:u16)
            n161 = Obtain Queue(element data type="") -> (queue out=w401:refnum<queue>)  [unwired: 4 in, 2 out]
            n162 = while "TCP-IP Listener" {
              tunnel: w395 -> [w425]
              tunnel: w401 -> [w420]
              stop <- w423 stop-if-true
              n163 = Dequeue Element(queue=w425) -> (queue out=w419:refnum<queue>, element=w418:T4, error out=w417:errorcluster)  [unwired: 2 in, 1 out]
              n164 = Unbundle By Name(w418) -> ("Cmd"=w422:string)
              n165 = case shown="Default" w422 {
                tunnel: [TRUE TRUE] -> w421
                tunnel: w420 -> [w432 _]
                tunnel: w419 -> [w430 _]
                tunnel: w418 -> [w429 _]
                tunnel: w417 -> [w428 _]
                tunnel: [w427 _] -> _
                tunnel: [w426 _] -> _
                frame Default {
                  # "If any command, stop listening\nRequeue command to be processed"
                  n166 = Enqueue Element(queue=w430, element=w429, error in (no error)=w428) -> (error out=w426:errorcluster)  [unwired: 1 in, 2 out]
                  n167 = Enqueue Element(queue=w432, element="Abort") -> (error out=w427:errorcluster)  [unwired: 2 in, 2 out]
                }
                frame "Connected" {
                  # "If connected, exit this loop"
                }
              }
              n168 = Unbundle By Name(w417) -> ("status"=w424:bool)
              n169 = Or(x=w421, y=w424) -> (x .or. y?=w423:bool)
            }
            n170 = property on="Status" class="Str"("Text.BGColor"=u32 16773632, "Value"="Listening" ("Status")) -> ()  [unwired: 2 in, 2 out]
            n171 = call "TCP-IP Mgr.Listener with Abort.vi"("Q.Abort"=w401, "port"=w400) -> ("error out"=w397:errorcluster, "Connected"=w398:bool, "Connection ID"=w399:refnum<k5>)  [unwired: 4 in, 3 out]
            n172 = Bundle By Name(cluster=w394, "TCPIP ID"=w399, "Connected"=w398) -> (w393:T13)
            n173 = case shown="False" w398 {
              tunnel: w395 -> [_ w414]
              tunnel: w397 -> [w405 _]
              tunnel: [w404 _] -> w396
              tunnel: w390 -> [_ w411]
              frame False {
                n174 = case shown="No Error" w405 {
                  selector: w405 -> [_ w410]
                  tunnel: [_ w410] -> w404
                  frame No Error {
                    n175 = property on="Status" class="Str"("Text.BGColor"=u32 13816530, "Value"="Idle" ("Status")) -> ()  [unwired: 2 in, 2 out]
                  }
                  frame Error {
                    n176 = property on="Status" class="Str"("Text.BGColor"=u32 16711680, "Value"="Error" ("Status")) -> ()  [unwired: 2 in, 2 out]
                  }
                }
              }
              frame True {
                n177 = call "Q.Enqueue Task.vi"("Task Name"="Read_Write" ("Cmd"), "Q In"=w414) -> ("error out"=w415:errorcluster)  [unwired: 8 in, 1 out]
                n178 = call "Q.Enqueue Task.vi"("Data1"=TRUE, "Error In"=w415, "Task Name"="Connect Event" ("Cmd"), "Q In"=w411) -> ()  [unwired: 6 in, 2 out]
              }
            }
          }
          frame "Connect" {
            n179 = Unbundle By Name(w440) -> ("Config.Listener"=w435:bool, "Config.IP"=w437:string, "Config.Port"=w436:u16)
            n180 = case shown="False" w435 {
              tunnel: [w459 _] -> w442
              tunnel: [w458 w482] -> w441
              tunnel: w440 -> [w454 w482]
              tunnel: w439 -> [w453 w480]
              tunnel: w438 -> [w452 _]
              tunnel: w437 -> [w448 _]
              tunnel: w436 -> [w447 _]
              frame False {
                n181 = TCP Open Connection(address=w448, remote port or service name=w447, timeout ms (60000)="Cnct Timeout") -> (connection ID=w445:refnum<k5>, error out=w446:errorcluster)  [unwired: 2 in]
                n182 = case shown="Error" w446 {
                  selector: w446 -> [_ w464]
                  tunnel: w445 -> [w461 _]
                  tunnel: [w461 _] -> w444
                  tunnel: [TRUE _] -> w457
                  tunnel: [_ w462] -> w456
                  frame No Error {
                  }
                  frame Error {
                    n183 = call <vilib>:"Clear Errors.vi"("error in (no error)"=w464, "specific error code to clear (0: all)"=56) -> ("error out"=w462:errorcluster)  [unwired: 4 in, 1 out]
                  }
                }
                n184 = property on="Status" class="Str"("Text.BGColor"=u32 16773632, "Value"="Connecting" ("Status")) -> (error out=w455:errorcluster)  [unwired: 2 in, 1 out]
                n185 = Bundle By Name(cluster=w454, "TCPIP ID"=w444, "Connected"=w457) -> (w458:T13)
                n186 = case shown="False" w457 {
                  tunnel: w453 -> [_ w477]
                  tunnel: [w472 _] -> w459
                  tunnel: w452 -> [w466 w475]
                  tunnel: w456 -> [w472 _]
                  tunnel: w455 -> [_ _]
                  tunnel: [w465 _] -> _
                  frame False {
                    n187 = To Variant(anything=FALSE) -> (Variant=w470:variant)
                    n188 = property on="Status" class="Str"("Text.BGColor"=u32 16711680, "Value"="Disconnected" ("Status")) -> ()  [unwired: 2 in, 2 out]
                    n189 = call "Q.Enqueue Task.vi"("Data1"=w470, "Task Name"="Connect Event" ("Cmd"), "Q In"=w466) -> ("error out"=w465:errorcluster)  [unwired: 7 in, 1 out]
                  }
                  frame True {
                    n190 = To Variant(anything=TRUE) -> (Variant=w474:variant)
                    n191 = call "Q.Enqueue Task.vi"("Task Name"="Read_Write" ("Cmd"), "Q In"=w477) -> ("error out"=w478:errorcluster)  [unwired: 8 in, 1 out]
                    n192 = call "Q.Enqueue Task.vi"("Data1"=w474, "Error In"=w478, "Task Name"="Connect Event" ("Cmd"), "Q In"=w475) -> ()  [unwired: 6 in, 2 out]
                  }
                }
              }
              frame True {
                n193 = call "Q.Enqueue Task.vi"("Task Name"="Listen" ("Cmd"), "Q In"=w480) -> ()  [unwired: 8 in, 2 out]
              }
            }
          }
          frame "Disconnect" {
            n194 = Unbundle By Name(w495) -> ("TCPIP ID"=w488:refnum<k5>)  [unwired: 1 out]
            n195 = TCP Close Connection(connection ID=w488) -> (error out=w487:errorcluster)  [unwired: 2 in, 1 out]
            n196 = call <vilib>:"Clear Errors.vi"("error in (no error)"=w487) -> ()  [unwired: 5 in, 2 out]
            n197 = Bundle By Name(cluster=w495, "TCPIP ID"=refnum<k5> refnum, "Connected"=FALSE) -> (w494:T13)
            n198 = To Variant(anything=FALSE) -> (Variant=w492:variant)
            n199 = property on="Status" class="Str"("Text.BGColor"=u32 16711680, "Value"="Disconnected" ("Status")) -> ()  [unwired: 2 in, 2 out]
            n200 = call "Q.Enqueue Task.vi"("Data1"=w492, "Task Name"="Connect Event" ("Cmd"), "Q In"=w484) -> ("error out"=w483:errorcluster)  [unwired: 7 in, 1 out]
            n201 = call <vilib>:"Clear Errors.vi"("error in (no error)"=w483) -> ()  [unwired: 5 in, 2 out]
          }
        }
      }
      frame "Error", Default {
        n202 = property on="Status" class="Str"("Text.BGColor"=u32 16711680, "Value"="Error" ("Status")) -> ()  [unwired: 2 in, 2 out]
        n203 = case shown="\"Error\"" w503 {
          selector: w503 -> [_ w513]
          tunnel: [w511 w514] -> _
          tunnel: w501 -> [_ _]
          tunnel: w502 -> [w512 _]
          tunnel: w505 -> [_ _]
          tunnel: w504 -> [_ _]
          tunnel: w497 -> [w510 _]
          frame "Error" {
            w508 = "Error" ("Cmd")
            # "Is a child.  Pass the error to the Parent Module"
            n204 = To Variant(anything=w512) -> (Variant=w507:variant)
            n205 = call "Q.Enqueue Item.vi"("Top of Q"=TRUE, "Data1"=w507, "Sub"=w508, "Cmd"=w508, "Q In"=w510) -> ("error out"=w511:errorcluster)  [unwired: 5 in, 1 out]
          }
          frame Default {
            n206 = Concatenate Strings("Undefined State: \"", w513, "\".") -> (w515:string)
            n207 = Bundle By Name(cluster=errorcluster {"status"=TRUE, "code"=-5000, "source"=""} ("error constant"), "source"=w515) -> (w514:errorcluster)
          }
        }
      }
      frame "Exit" {
        n208 = Unbundle By Name(w519) -> ("TCPIP ID"=w520:refnum<k5>)
        n209 = TCP Close Connection(connection ID=w520) -> (error out=w521:errorcluster)  [unwired: 2 in, 1 out]
        n210 = call <vilib>:"Clear Errors.vi"("error in (no error)"=w521) -> ()  [unwired: 5 in, 2 out]
      }
    }
  }
